vi "weight projected images.vi"(6 "reset?":bool, 7 "weight":dbl, 10 "projections":T2) -> (2 "projections out":T1, 4 "in loop reset":bool, 5 "reset":bool)   [LabVIEW 2010]
panel:
  out "Numeric":i32
  out "ch1 sum":u32
  out "ch0 sum":u32
  # "double precision on input lets averaging go over parts of pixels -- important"
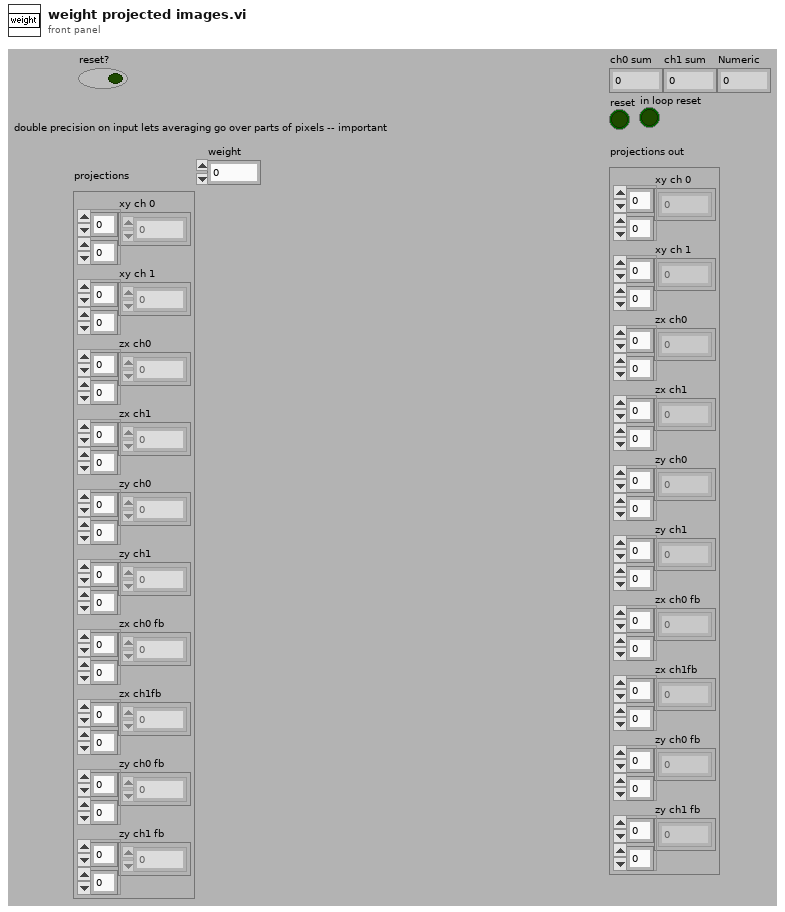
[diagram p1: front panel]
types:
  T1 = cluster{"xy ch 0":u16[][], "xy ch 1":u16[][], "zx ch0":u16[][], "zx ch1":u16[][], "zy ch0":u16[][], "zy ch1":u16[][], "zx ch0 fb":u16[][], "zx ch1fb":u16[][], "zy ch0 fb":u16[][], "zy ch1 fb":u16[][]}
  T2 = cluster{"xy ch 0":dbl[][], "xy ch 1":dbl[][], "zx ch0":dbl[][], "zx ch1":dbl[][], "zy ch0":dbl[][], "zy ch1":dbl[][], "zx ch0 fb":dbl[][], "zx ch1fb":dbl[][], "zy ch0 fb":dbl[][], "zy ch1 fb":dbl[][]}
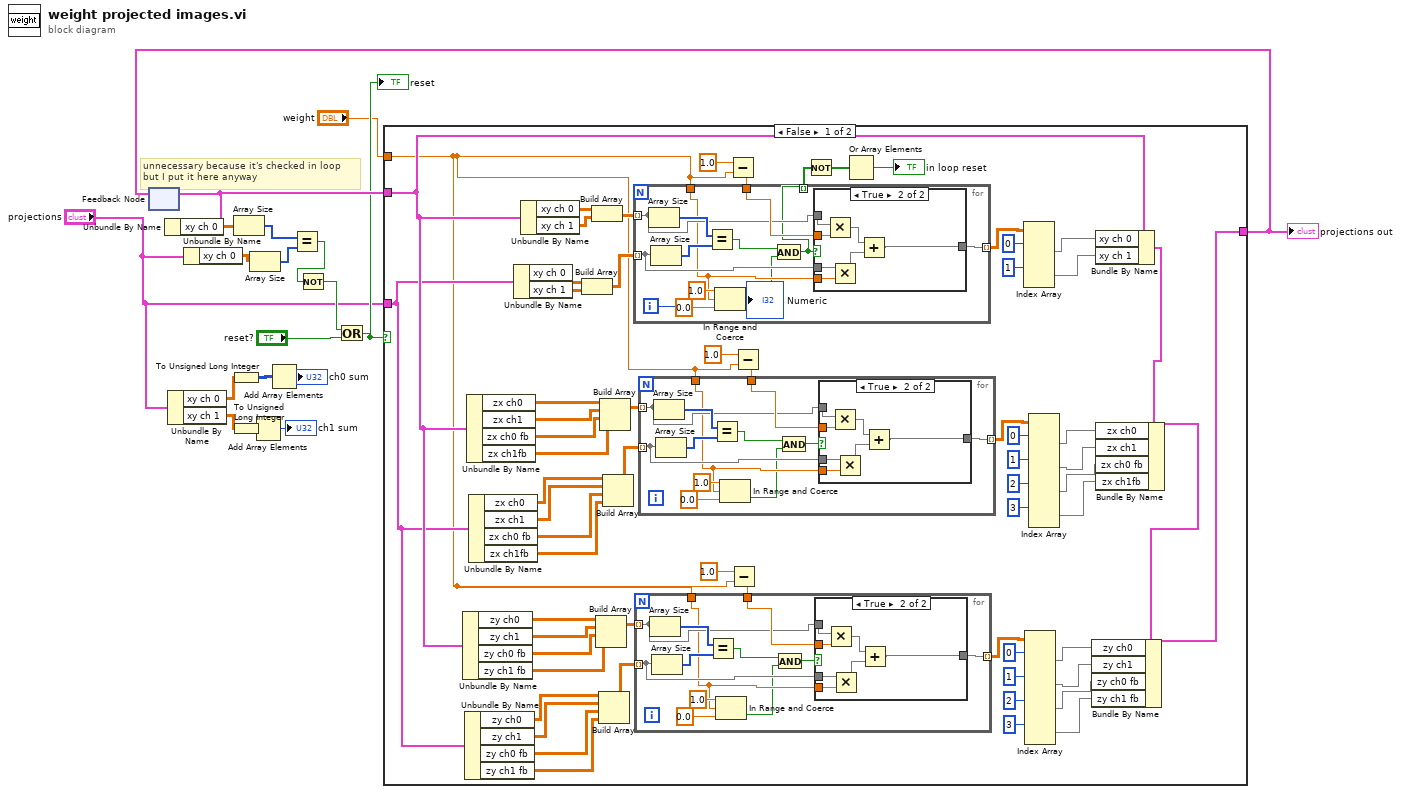
[diagram p0: block diagram]
diagram:
  # "unnecessary because it's checked in loop\nbut I put it here anyway"
  n1 = feedback #1() -> (w17:T2)  [unwired: 1 in]
  n2 = Unbundle By Name(w17) -> ("xy ch 0"=w15:dbl[][])
  n3 = Unbundle By Name("projections") -> ("xy ch 0"=w8:dbl[][], "xy ch 1"=w6:dbl[][])
  n4 = Unbundle By Name("projections") -> ("xy ch 0"=w16:dbl[][])
  n5 = To Unsigned Long Integer(number=w8) -> (unsigned 32bit integer=w5:u32[][])
  n6 = To Unsigned Long Integer(number=w6) -> (unsigned 32bit integer=w4:u32[][])
  n7 = Array Size(array=w15) -> (size(s)=w14:i32[])
  n8 = Array Size(array=w16) -> (size(s)=w13:i32[])
  n9 = Add Array Elements(numeric array=w4) -> (sum=→"ch1 sum":u32)
  n10 = Add Array Elements(numeric array=w5) -> (sum=→"ch0 sum":u32)
  n11 = Equal?(x=w14, y=w13) -> (x = y?=w12:bool)
  n12 = Not(x=w12) -> (.not. x?=w10:bool)
  n13 = Or(x=w10, y="reset?") -> (x .or. y?=w11:bool)
  "reset" <- w11
  n14 = case shown="False" w11 {
    tunnel: "projections" -> [w25 w144]
    tunnel: [w23 w144] -> w1
    tunnel: w17 -> [w26 _]
    tunnel: "weight" -> [w22 _]
    frame False {
      n15 = Unbundle By Name(w26) -> ("zy ch0"=w34:dbl[][], "zy ch1"=w33:dbl[][], "zy ch0 fb"=w30:dbl[][], "zy ch1 fb"=w29:dbl[][])
      n16 = Unbundle By Name(w25) -> ("zy ch0"=w32:dbl[][], "zy ch1"=w31:dbl[][], "zy ch0 fb"=w28:dbl[][], "zy ch1 fb"=w27:dbl[][])
      n17 = Unbundle By Name(w26) -> ("zx ch0"=w56:dbl[][], "zx ch1"=w55:dbl[][], "zx ch0 fb"=w51:dbl[][], "zx ch1fb"=w50:dbl[][])
      n18 = Unbundle By Name(w25) -> ("zx ch0"=w54:dbl[][], "zx ch1"=w53:dbl[][], "zx ch0 fb"=w49:dbl[][], "zx ch1fb"=w48:dbl[][])
      n19 = Unbundle By Name(w25) -> ("xy ch 0"=w71:dbl[][], "xy ch 1"=w70:dbl[][])
      n20 = Unbundle By Name(w26) -> ("xy ch 0"=w73:dbl[][], "xy ch 1"=w72:dbl[][])
      n21 = Build Array(w71, w70) -> (w81:dbl[][][])
      n22 = Build Array(w73, w72) -> (w82:dbl[][][])
      n23 = Build Array(w34, w33, w30, w29) -> (w47:dbl[][][])
      n24 = Build Array(w32, w31, w28, w27) -> (w46:dbl[][][])
      n25 = Build Array(w56, w55, w51, w50) -> (w69:dbl[][][])
      n26 = Build Array(w54, w53, w49, w48) -> (w68:dbl[][][])
      n27 = Subtract(x=1.0, y=w22) -> (x-y=w79:dbl)
      n28 = for {
        tunnel: w82 -> [w130] mode=indexing
        tunnel: w81 -> [w131] mode=indexing
        tunnel: w22 -> [w127]
        tunnel: w79 -> [w133]
        tunnel: [w132] -> w78 mode=indexing
        tunnel: [w124] -> w21 mode=indexing
        i -> [w123]
        n29 = Array Size(array=w130) -> (size(s)=w134:i32[])
        n30 = Array Size(array=w131) -> (size(s)=w135:i32[])
        n31 = Equal?(x=w134, y=w135) -> (x = y?=w125:bool)
        n32 = In Range and Coerce(upper limit=1.0, x=w127, lower limit=0.0) -> (In Range?=w126:bool)  [unwired: 1 out]
        n33 = And(x=w125, y=w126) -> (x .and. y?=w124:bool)
        n34 = case shown="True" w124 {
          tunnel: w131 -> [w136 w142]
          tunnel: w130 -> [_ w143]
          tunnel: w127 -> [_ w141]
          tunnel: w133 -> [_ w140]
          tunnel: [w136 w137] -> w132
          frame False {
          }
          frame True {
            n35 = Multiply(x=w143, y=w140) -> (x*y=w139:dbl[][])
            n36 = Multiply(x=w142, y=w141) -> (x*y=w138:dbl[][])
            n37 = Add(x=w139, y=w138) -> (x+y=w137:dbl[][])
          }
        }
        "Numeric" <- w123
      }
      n38 = Subtract(x=1.0, y=w22) -> (x-y=w44:dbl)
      n39 = for {
        tunnel: w47 -> [w89] mode=indexing
        tunnel: w46 -> [w90] mode=indexing
        tunnel: w22 -> [w86]
        tunnel: w44 -> [w92]
        tunnel: [w91] -> w43 mode=indexing
        n40 = Array Size(array=w89) -> (size(s)=w93:i32[])
        n41 = Array Size(array=w90) -> (size(s)=w94:i32[])
        n42 = Equal?(x=w93, y=w94) -> (x = y?=w83:bool)
        n43 = In Range and Coerce(upper limit=1.0, x=w86, lower limit=0.0) -> (In Range?=w84:bool)  [unwired: 1 out]
        n44 = And(x=w83, y=w84) -> (x .and. y?=w85:bool)
        n45 = case shown="True" w85 {
          tunnel: w90 -> [w95 w101]
          tunnel: w89 -> [_ w102]
          tunnel: w86 -> [_ w100]
          tunnel: w92 -> [_ w99]
          tunnel: [w95 w96] -> w91
          frame False {
          }
          frame True {
            n46 = Multiply(x=w102, y=w99) -> (x*y=w98:dbl[][])
            n47 = Multiply(x=w101, y=w100) -> (x*y=w97:dbl[][])
            n48 = Add(x=w98, y=w97) -> (x+y=w96:dbl[][])
          }
        }
      }
      n49 = Subtract(x=1.0, y=w22) -> (x-y=w66:dbl)
      n50 = for {
        tunnel: w69 -> [w109] mode=indexing
        tunnel: w68 -> [w110] mode=indexing
        tunnel: w22 -> [w106]
        tunnel: w66 -> [w112]
        tunnel: [w111] -> w65 mode=indexing
        n51 = Array Size(array=w109) -> (size(s)=w113:i32[])
        n52 = Array Size(array=w110) -> (size(s)=w114:i32[])
        n53 = Equal?(x=w113, y=w114) -> (x = y?=w103:bool)
        n54 = In Range and Coerce(upper limit=1.0, x=w106, lower limit=0.0) -> (In Range?=w104:bool)  [unwired: 1 out]
        n55 = And(x=w103, y=w104) -> (x .and. y?=w105:bool)
        n56 = case shown="True" w105 {
          tunnel: w110 -> [w115 w121]
          tunnel: w109 -> [_ w122]
          tunnel: w106 -> [_ w120]
          tunnel: w112 -> [_ w119]
          tunnel: [w115 w116] -> w111
          frame False {
          }
          frame True {
            n57 = Multiply(x=w122, y=w119) -> (x*y=w118:dbl[][])
            n58 = Multiply(x=w121, y=w120) -> (x*y=w117:dbl[][])
            n59 = Add(x=w118, y=w117) -> (x+y=w116:dbl[][])
          }
        }
      }
      n60 = Not(x=w21) -> (.not. x?=w19:bool[])
      n61 = Or Array Elements(Boolean array=w19) -> (logical OR=→"in loop reset":bool)
      n62 = Index Array(array=w78, index (dim 0) #1=0 ("index (row)"), index (dim 0) #2=1 ("index (page)")) -> (element #1=w75:dbl[][], element #2=w74:dbl[][])  [unwired: 4 in]
      n63 = Index Array(array=w43, index (dim 0) #1=0 ("index (row)"), index (dim 0) #2=1 ("index (page)"), index (dim 0) #3=2 ("index (page)"), index (dim 0) #4=3 ("index (page)")) -> (element #1=w38:dbl[][], element #2=w37:dbl[][], element #3=w36:dbl[][], element #4=w35:dbl[][])  [unwired: 8 in]
      n64 = Index Array(array=w65, index (dim 0) #1=0 ("index (row)"), index (dim 0) #2=1 ("index (page)"), index (dim 0) #3=2 ("index (page)"), index (dim 0) #4=3 ("index (page)")) -> (element #1=w60:dbl[][], element #2=w59:dbl[][], element #3=w58:dbl[][], element #4=w57:dbl[][])  [unwired: 8 in]
      n65 = Bundle By Name(cluster=w26, "xy ch 0"=w75, "xy ch 1"=w74) -> (w52:T2)
      n66 = Bundle By Name(cluster=w52, "zx ch0"=w60, "zx ch1"=w59, "zx ch0 fb"=w58, "zx ch1fb"=w57) -> (w24:T2)
      n67 = Bundle By Name(cluster=w24, "zy ch0"=w38, "zy ch1"=w37, "zy ch0 fb"=w36, "zy ch1 fb"=w35) -> (w23:T2)
    }
    frame True {
    }
  }
  "projections out" <- w1
  n68 = feedback-in #1(w1) -> ()
